vi "Initialize.vi"(8 "error in (no error)":errorcluster) -> (0 "error out":errorcluster, 3 "Power Meter out":refnum<class "Power Meter.lvclass">)   [LabVIEW 2009, in "Power Meter.lvclass"]
doc: "Initializes the Power Meter."
uses:
  Power Meter.lvclass
panel:
  in  "Local Lockout (0:1)":u32(ring) items=["Off", "On"]
  in  "ATTN (0:1)":u32(ring) items=["Off", "On"]
  in  "Run/Stop (1:0)":u32(ring)=1 items=["Stop", "Run"]
  in  "AVG (1:3)":u32(ring)=2 items=["Slow"=1, "Medium"=2, "Fast"=3]
  in  "Units (1:4)":u32(ring)=1 items=["W"=1, "dB"=2, "dBm"=3, "REL"=4]
  in  "Zero (0:1)":u32(ring) items=["Off", "On"]
  in  "Beeper (0:1)":u32(ring) items=["Off", "On"]
  in  "Backlight (0:2)":u32(ring)=1 items=["Off", "Low", "High"]
  in  "Range (0-Auto,1:8)":u32(ring) items=["Auto", "Lowest", "2", "3", "4", "5", "6", "7", "Highest"]
  in  "Wavelength (nnnn)":dbl[unit]=8.210000000000001e-07
  in  "Set":bool
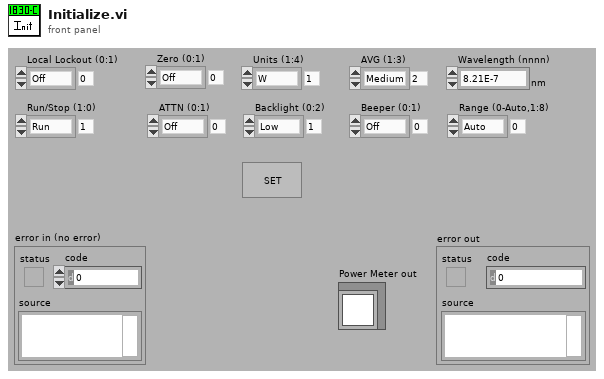
[diagram p1: front panel]
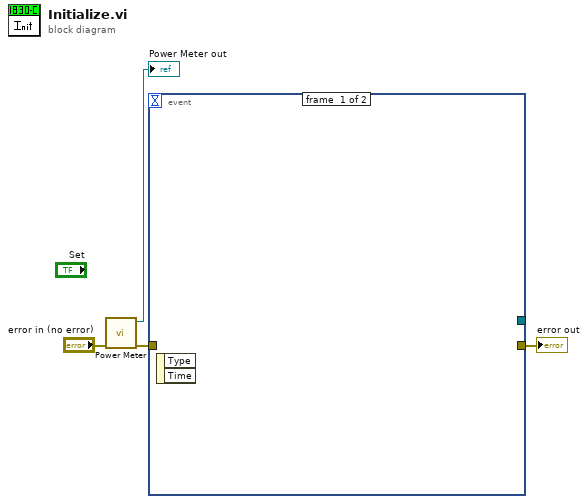
[diagram p0: block diagram]
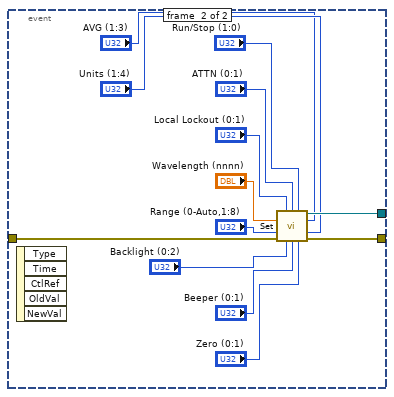
[diagram p2: hidden frame]
diagram:
  n1 = call "Power Meter.vi"("error in (no error)"="error in (no error)") -> ("error out"=w3:errorcluster, "Power Meter out"=→"Power Meter out":refnum<class "Power Meter.lvclass">)  [unwired: 9 in]
  n2 = event shown="[1] \"Set\": Value Change" {
    selector: _ -> [_ _]
    dyn-events: _ -> [_ _]
    timeout: _ -> [_ _]
    tunnel: [_ w17] -> _
    tunnel: w3 -> [_ w14]
    tunnel: [_ w10] -> w2
    event #0 {
      n3 = event-data() -> ()  [unwired: 1 in, 2 out]
    }
    event #1 {
      n4 = event-data() -> ()  [unwired: 1 in, 5 out]
      n5 = call "Set.vi"("Local Lockout (0:1)"="Local Lockout (0:1)", "ATTN (0:1)"="ATTN (0:1)", "Run/Stop (1:0)"="Run/Stop (1:0)", "Wavelength (nnnn)"="Wavelength (nnnn)", "AVG (1:3)"="AVG (1:3)", "Range (0-Auto,1:8)"="Range (0-Auto,1:8)", "Units (1:4)"="Units (1:4)", "error in (no error)"=w14, "Backlight (0:2)"="Backlight (0:2)", "Beeper (0:1)"="Beeper (0:1)", "Zero (0:1)"="Zero (0:1)") -> ("VISA resource name out"=w17:refnum<visa-resource-name>, "error out"=w10:errorcluster)  [unwired: 3 in]
    }
  }
  "error out" <- w2
